vi "CreatePublicEvents.vi"(8 "error in (no error)":errorcluster, 11 "DisplayWaveforms":refnum<class "DisplayWaveforms.lvclass">) -> (0 "error out":errorcluster, 3 "DisplayWaveforms out":refnum<class "DisplayWaveforms.lvclass">)   [LabVIEW 2018, in "DisplayWaveform.lvlib" / "DisplayWaveforms.lvclass"]
doc: "---------------------------------------------------------------\nJKI State Machine Objects™\nhttp://jki.net/state-machine-objects/\nCopyright (C) 2005-2015, JKI <info@jki.net>\nALL RIGHTS RESERVEDJKI State Machine Objects (SMO) 1.0.0.5\nJKI - JKI\nCopyright (c) 2016, JKI"
uses:
  DisplayWaveforms.lvclass
  <vilib>/JKI/JKI SMO/SMO.UI/SMO.UI.lvclass
panel:
  # "For instructions on how to use the JKI State Machine Objects, examples and video tutorials, visit:\nhttp://jki.net/state-machine-objects/\n\nJKI State Machine Objects™\nhttp://jki.net/state-machine-objects/\nCopyright (C) 2005-2015, JKI <info@jki.net>\nALL RIGHTS RESERVED"
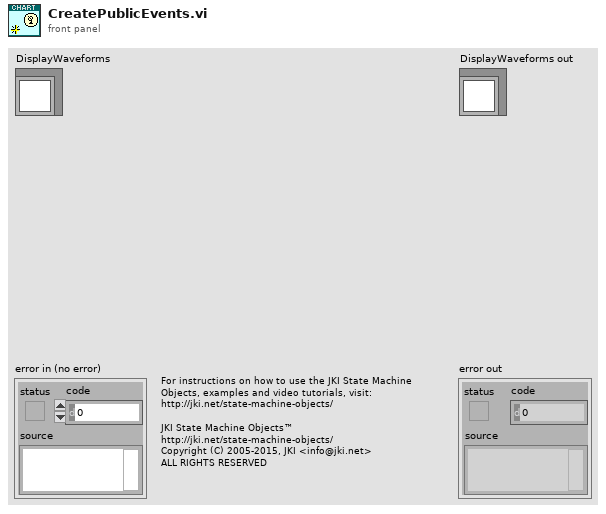
[diagram p1: front panel]
types:
  T1 = typedef "DisplayWaveform.lvlib/DisplayWaveforms.lvclass/PrivateData--Ref.ctl" = refnum<data-value>
  T2 = typedef "DisplayWaveform.lvlib/DisplayWaveforms.lvclass/PrivateData--Cluster.ctl" = cluster{"Public Events":T3, "Protected Events":T4, "Data":string, "Dependencies":T5}
  T3 = typedef "DisplayWaveform.lvlib/DisplayWaveforms.lvclass/PublicEvents--Cluster.ctl" = cluster{"Chart Cleared":refnum<user-event>, "Chart Exported":refnum<user-event>, "ChartParams Set":refnum<user-event>}
  T4 = typedef "DisplayWaveform.lvlib/DisplayWaveforms.lvclass/ProtectedEvents--Cluster.ctl" = cluster{"Clear Chart":refnum<user-event>, "Pause Chart":refnum<user-event>, "Update Chart":refnum<user-event>, "Export Chart":refnum<user-event>, "Set ChartParams":refnum<user-event>}
  T5 = typedef "DisplayWaveform.lvlib/DisplayWaveforms.lvclass/Dependencies--Cluster.ctl" = cluster{"New Value":refnum<user-event>}
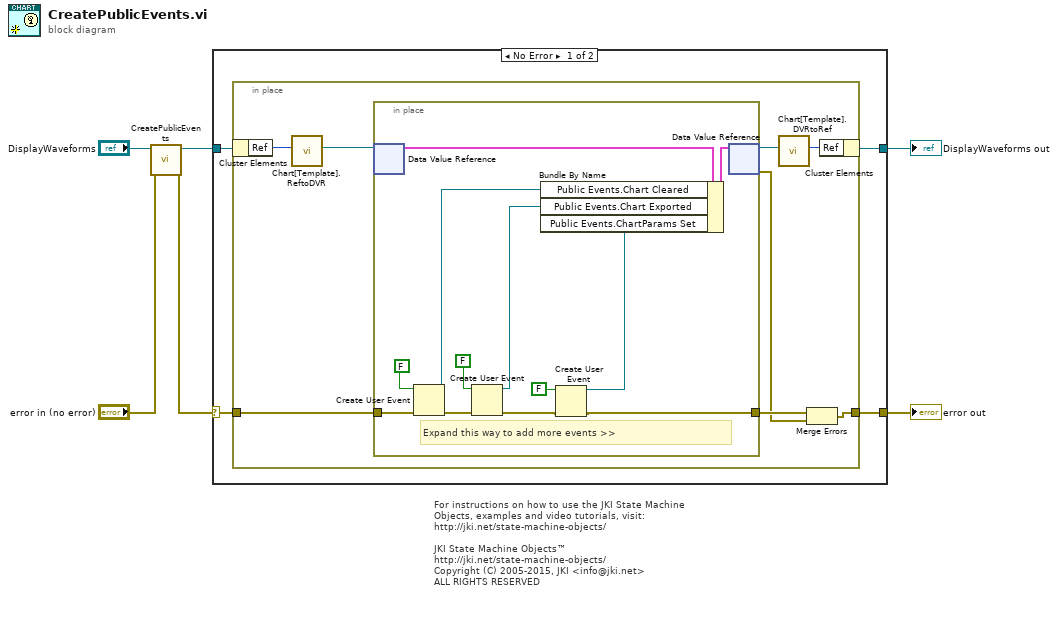
[diagram p0: block diagram]
diagram:
  # "For instructions on how to use the JKI State Machine Objects, examples and video tutorials, visit:\nhttp://jki.net/state-machine-objects/\n\nJKI State Machine Objects™\nhttp://jki.net/state-machine-objects/\nCopyright (C) 2005-2015, JKI <info@jki.net>\nALL RIGHTS RESERVED"
  n1 = call-parent "CreatePublicEvents.vi"("error in (no error)"="error in (no error)", "SMO.UI"="DisplayWaveforms") -> ("error out"=w1:errorcluster, "SMO.UI out"=w3:refnum<class "DisplayWaveforms.lvclass">)  [unwired: 8 in]
  n2 = case shown="No Error" w1 {
    selector: w1 -> [w8 w32]
    tunnel: [w7 w32] -> w5
    tunnel: [w9 w31] -> w6
    tunnel: w3 -> [w10 w31]
    frame No Error {
      n3 = in-place {
        in-place-border: w8 -> [w18]
        in-place-border: [w15] -> w7
        n4 = in-place-cluster #1(w10) -> ("Ref"=w14:u32)
        n5 = call "Chart[Template].ReftoDVR.vi"("Ref"=w14) -> ("Ref"=w13:T1)  [unwired: 10 in]
        n6 = in-place {
          in-place-border: w18 -> [w28]
          in-place-border: [w19] -> w17
          # "Expand this way to add more events >>"
          n7 = in-place-dvr #2(w13) -> (w29:T2)  [unwired: 1 out]
          n8 = Create User Event(user event datatype=FALSE ("Boolean"), error in=w28) -> (user event=w26:refnum<user-event>, error out=w25:errorcluster)
          n9 = Create User Event(user event datatype=FALSE ("Boolean"), error in=w25) -> (user event=w24:refnum<user-event>, error out=w22:errorcluster)
          n10 = Create User Event(user event datatype=FALSE ("Boolean"), error in=w22) -> (user event=w20:refnum<user-event>, error out=w19:errorcluster)
          n11 = Bundle By Name(cluster=w29, "Public Events.Chart Cleared"=w26, "Public Events.Chart Exported"=w24, "Public Events.ChartParams Set"=w20) -> (w30:T2)
          n12 = in-place-dvr #2(w30) -> (w12:T1, w16:errorcluster)
        }
        n13 = call "Chart[Template].DVRtoRef.vi"("Ref"=w12) -> ("Ref"=w11:u32)  [unwired: 10 in]
        n14 = Merge Errors(w17, w16) -> (w15:errorcluster)
        n15 = in-place-cluster #1("Ref"=w11) -> (w9:refnum<class "DisplayWaveforms.lvclass">)
      }
    }
    frame Error {
    }
  }
  "error out" <- w5
  "DisplayWaveforms out" <- w6
